vi "SensorInterrupt.vi"(8 "error in (no error)":errorcluster, 11 "Drive in":refnum<class "Drive.lvclass">) -> (0 "error out":errorcluster, 3 "Drive out":refnum<class "Drive.lvclass">)   [LabVIEW 2017, in "Drive.lvclass"]
uses:
  Drive.lvclass
  Subsystem.lvclass
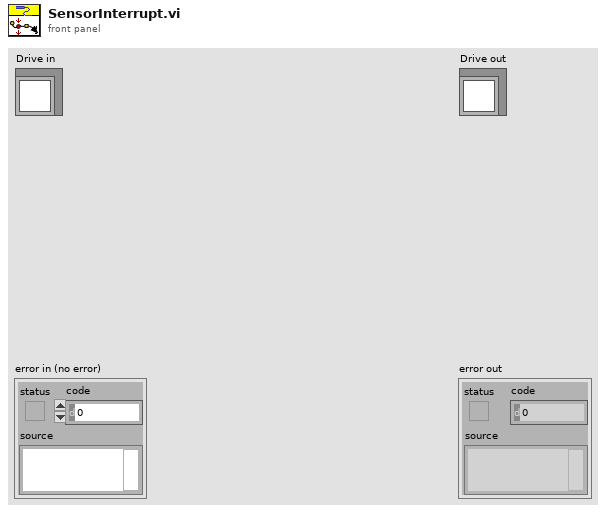
[diagram p1: front panel]
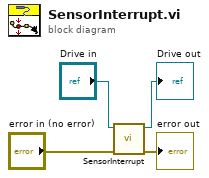
[diagram p0: block diagram]
diagram:
  n1 = call-parent "SensorInterrupt.vi"("error in (no error)"="error in (no error)", "Subsystem in"="Drive in") -> ("error out"=→"error out":errorcluster, "Subsystem out"=→"Drive out":refnum<class "Drive.lvclass">)  [unwired: 8 in]
